vi "json_indentlevel.vi"(7 "indent level":i32, 10 "string":string) -> (2 "indented string":string)   [LabVIEW 2020, in "Caraya.lvlib" / "Test Result.lvclass"]
uses:
  Test Result.lvclass
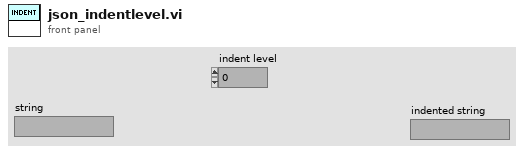
[diagram p1: front panel]
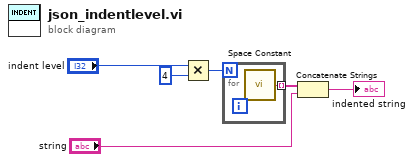
[diagram p0: block diagram]
diagram:
  n1 = Multiply(x="indent level", y=4) -> (x*y=w6:i32)
  n2 = for {
    N: w6 -> [_]
    tunnel: [w7] -> w2 mode=indexing
    n3 = call <vilib>:"Space Constant.vi"() -> ("String"=w7:string)
  }
  n4 = Concatenate Strings(w2, "string") -> (→"indented string":string)
